vi "读取bmp图片.vi"(0 "path to BMP file":path caption="BMP文件路径") -> (4 "图像归一化二维数组":dbl[][](array[numeric]) caption="8位像素图", 6 "图像行":i32, 8 "图像列":i32)   [LabVIEW 2018]
panel:
  out "原图":u8[][](graph)
  out "原图像":picture
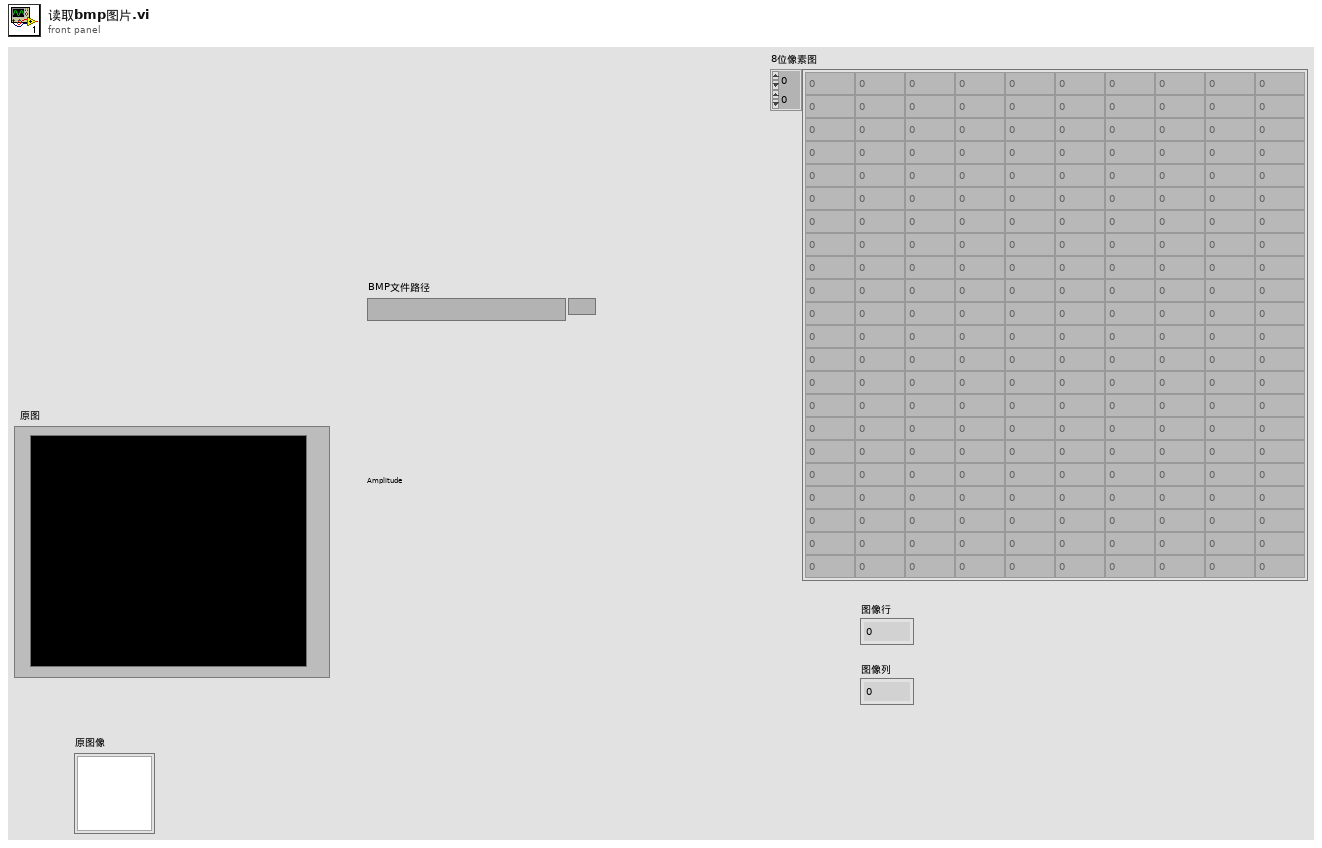
[diagram p1: front panel]
types:
  T1 = typedef "imagedata.ctl" = cluster{"image type":i32, "image depth":i32, "image":u8[], "mask":u8[], "colors":u32[], "Rectangle":cluster{"left":i16, "top":i16, "right":i16, "bottom":i16}}
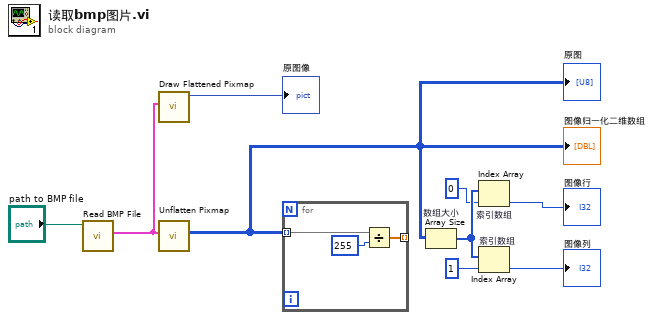
[diagram p0: block diagram]
diagram:
  n1 = call <vilib>:"Read BMP File.vi"("path to BMP file"="path to BMP file") -> ("image data"=w8:T1)  [unwired: 8 in, 2 out]
  n2 = call <vilib>:"Draw Flattened Pixmap.vi"("image data"=w8) -> ("new picture"=→"原图像":picture)  [unwired: 8 in]
  n3 = call <vilib>:"Unflatten Pixmap.vi"("image data"=w8) -> ("8-bit pixmap"=w1:u8[][])  [unwired: 10 out]
  "原图" <- w1
  "图像归一化二维数组" <- w1
  n4 = for {
    tunnel: w1 -> [w12] mode=indexing
    tunnel: [w10] -> _ mode=indexing
    n5 = Divide(x=w12, y=255) -> (x/y=w10:dbl[])
  }
  n6 = Array Size "数组大小"(array=w1) -> (size(s)=w7:i32[])
  n7 = Index Array "索引数组"(array=w7, index=0) -> (element=→"图像行":i32)
  n8 = Index Array "索引数组"(array=w7, index=1) -> (element=→"图像列":i32)
